vi "calc_error_OD.vi"(8 "error in (no error)":errorcluster, 10 "OD":dbl[](array[numeric]), 11 "Detector in":refnum<class "Detector.lvclass">) -> (0 "error out":errorcluster, 3 "Detector out":refnum<class "Detector.lvclass">)   [LabVIEW 2018, in "Detector.lvclass"]
uses:
  Detector.lvclass
  Detector.lvclass/Detector.ctl
  <vilib>/Analysis/NI_AALBase.lvlib
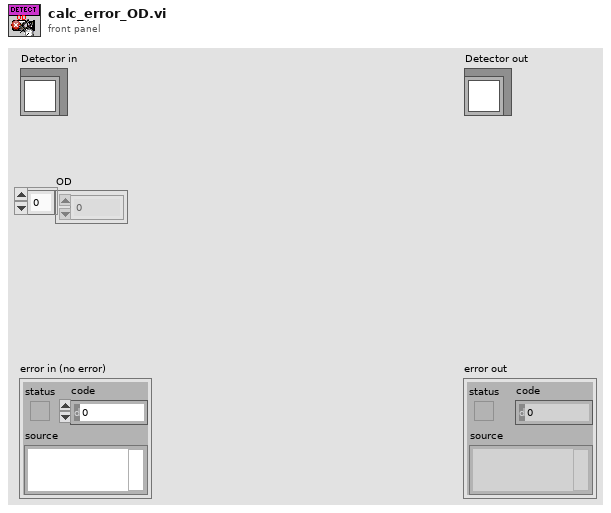
[diagram p1: front panel]
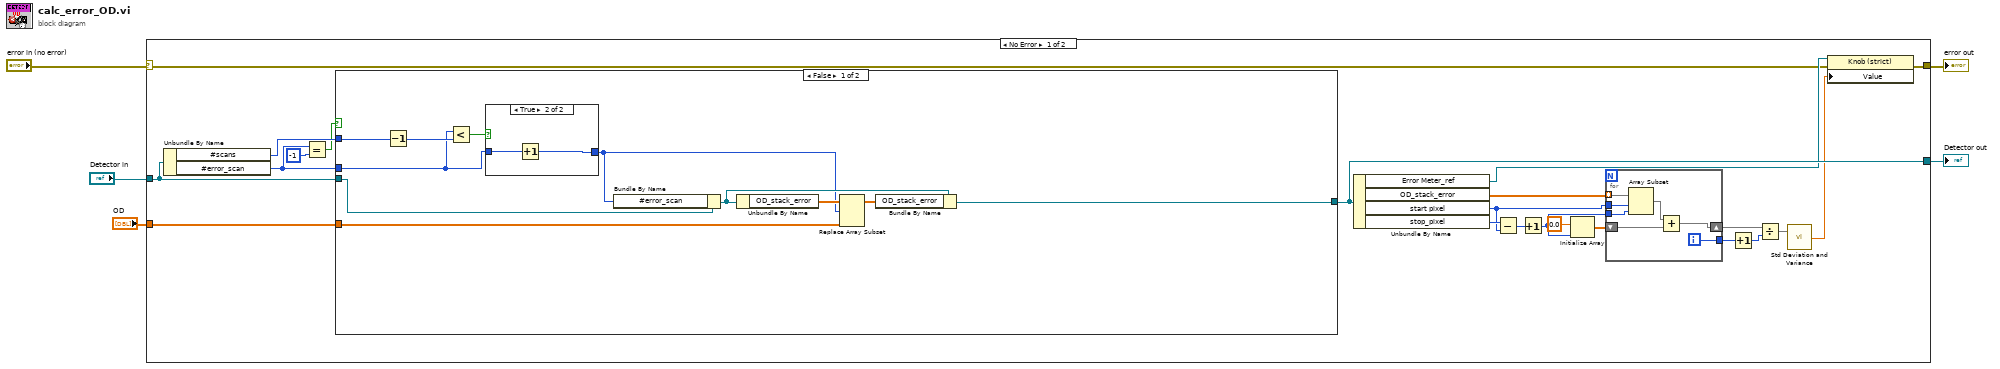
[diagram p0: block diagram]
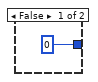
[diagram p2: hidden frame]
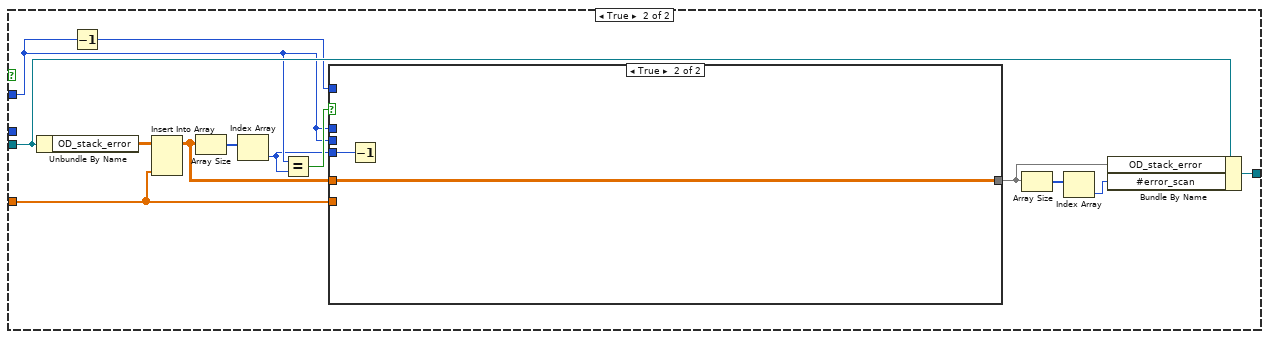
[diagram p3: hidden frame]
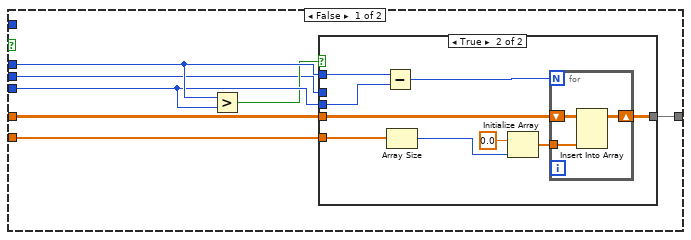
[diagram p4: hidden frame]
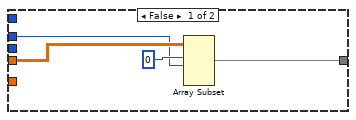
[diagram p5: hidden frame]
diagram:
  n1 = case shown="No Error" "error in (no error)" {
    selector: "error in (no error)" -> [w7 w88]
    tunnel: [w15 w88] -> w4
    tunnel: [w23 w87] -> w2
    tunnel: "Detector in" -> [w14 w87]
    tunnel: "OD" -> [w6 _]
    frame No Error {
      n2 = Unbundle By Name(w14) -> ("#scans"=w27:i32, "#error_scan"=w26:i32)
      n3 = Equal?(x=w26, y=-1) -> (x = y?=w24:bool)
      n4 = case shown="False" w24 {
        tunnel: w14 -> [w41 w60]
        tunnel: [w36 w59] -> w23
        tunnel: w6 -> [w38 w56]
        tunnel: w27 -> [w45 w53]
        tunnel: w26 -> [w42 _]
        frame False {
          n5 = Decrement(x=w45) -> (x-1=w44:i32)
          n6 = Less?(x=w42, y=w44) -> (x < y?=w43:bool)
          n7 = case shown="True" w43 {
            tunnel: w42 -> [_ w48]
            tunnel: [0 w47] -> w35
            frame False {
            }
            frame True {
              n8 = Increment(x=w48) -> (x+1=w47:i32)
            }
          }
          n9 = Bundle By Name(cluster=w41, "#error_scan"=w35) -> (w37:refnum<class "Detector.lvclass">)
          n10 = Unbundle By Name(w37) -> ("OD_stack_error"=w40:dbl[][])
          n11 = Replace Array Subset(array=w40, new element=w38, index (row)=w35) -> (w39:dbl[][])  [unwired: 1 in]
          n12 = Bundle By Name(cluster=w37, "OD_stack_error"=w39) -> (w36:refnum<class "Detector.lvclass">)
        }
        frame True {
          n13 = Unbundle By Name(w60) -> ("OD_stack_error"=w61:dbl[][])
          n14 = Decrement(x=w53) -> (x-1=w55:i32)
          n15 = Insert Into Array(array=w61, new element=w56) -> (w57:dbl[][])  [unwired: 2 in]
          n16 = Array Size(array=w57) -> (size(s)=w58:i32[])
          n17 = Index Array(array=w58) -> (element=w52:i32)  [unwired: 1 in]
          n18 = Equal?(x=w53, y=w52) -> (x = y?=w54:bool)
          n19 = case shown="True" w54 {
            tunnel: w57 -> [w68 w86]
            tunnel: [w67 w86] -> w50
            tunnel: w56 -> [w66 _]
            tunnel: w55 -> [_ _]
            tunnel: w53 -> [w65 _]
            tunnel: w52 -> [w64 w85]
            tunnel: w53 -> [w62 _]
            frame False {
              n20 = Greater?(x=w65, y=w64) -> (0:w63:bool)
              n21 = case shown="True" w63 {
                tunnel: w68 -> [w72 w81]
                tunnel: [w71 w80] -> w67
                tunnel: w66 -> [_ w79]
                tunnel: w65 -> [_ w75]
                tunnel: w64 -> [_ w74]
                tunnel: w62 -> [w69 _]
                frame False {
                  n22 = Array Subset(array=w72, index (row)=0 ("index"), length (row)=w69) -> (w71:dbl[][])  [unwired: 2 in]
                }
                frame True {
                  n23 = Subtract(x=w75, y=w74) -> (x-y=w73:i32)
                  n24 = Array Size(array=w79) -> (size(s)=w77:i32)
                  n25 = Initialize Array(0.0 ("dimension size"), w77) -> (w76:dbl[])
                  n26 = for {
                    N: w73 -> [_]
                    shift-right: [w83] -> w80
                    shift-left: w81 -> [w84]
                    tunnel: w76 -> [w82]
                    n27 = Insert Into Array(array=w84, new element=w82) -> (w83:dbl[][])  [unwired: 2 in]
                  }
                }
              }
            }
            frame True {
              n28 = Decrement(x=w85) -> ()  [unwired: 1 out]
            }
          }
          n29 = Array Size(array=w50) -> (size(s)=w51:i32[])
          n30 = Index Array(array=w51) -> (element=w49:i32)  [unwired: 1 in]
          n31 = Bundle By Name(cluster=w60, "OD_stack_error"=w50, "#error_scan"=w49) -> (w59:refnum<class "Detector.lvclass">)
        }
      }
      n32 = Unbundle By Name(w23) -> ("Error Meter_ref"=w17:refnum<vi>, "OD_stack_error"=w22:dbl[][], "start pixel"=w9:i32, "stop_pixel"=w10:i32)
      n33 = Subtract(x=w10, y=w9) -> (x-y=w13:i32)
      n34 = Increment(x=w13) -> (x+1=w8:i32)
      n35 = Initialize Array(0.0 ("element"), w8) -> (w11:dbl[])
      n36 = for {
        shift-right: [w34] -> w21
        shift-left: w11 -> [w29]
        tunnel: w22 -> [w32] mode=indexing
        tunnel: [w33] -> w20
        tunnel: w9 -> [w31]
        tunnel: w8 -> [w30]
        i -> [w33]
        n37 = Array Subset(array=w32, index=w31, length=w30) -> (w28:dbl[])
        n38 = Add(x=w28, y=w29) -> (x+y=w34:dbl[])
      }
      n39 = Increment(x=w20) -> (x+1=w19:i32)
      n40 = Divide(x=w21, y=w19) -> (x/y=w18:dbl[])
      n41 = call <vilib>:"Std Deviation and Variance.vi"("X"=w18) -> ("standard deviation"=w16:dbl)  [unwired: 1 in, 2 out]
      n42 = property class="Knob (strict)"(reference=w17, error in=w7, "Value"=w16) -> (error out=w15:errorcluster)  [unwired: 1 out]
    }
    frame Error {
    }
  }
  "error out" <- w4
  "Detector out" <- w2
